vi "OPC Read Bool Variables.vi"() -> ()   [LabVIEW 2016]
uses:
  Architecture/Queue Management/ARC_Queue Valid.vi
panel:
  out "本地/远程":bool
  out "主电机准备好":bool
  out "主电机故障":bool
  out "主电机运行":bool
  out "变频器合闸":bool
  in  "Caller":string
  out "介质阀":bool
  out "增压1":bool
  out "排气1":bool
  out "进介质2":bool
  out "进介质1":bool
  out "增压2":bool
  out "排气2":bool
  out "调节阀电源":bool
  out "流量计电源":bool
  out "急停":bool
  out "容器间":bool
  out "球阀开":bool
  out "球阀关":bool
  out "油冷机故障":bool
  out "油冷机运行":bool
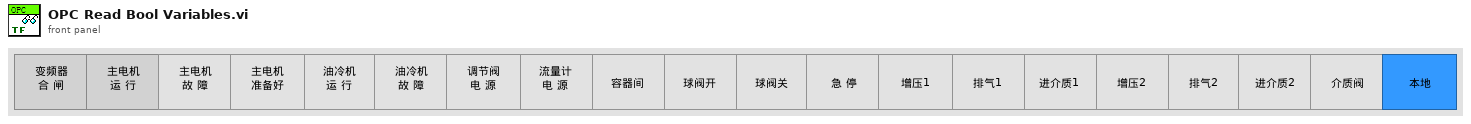
[diagram p1: front panel]
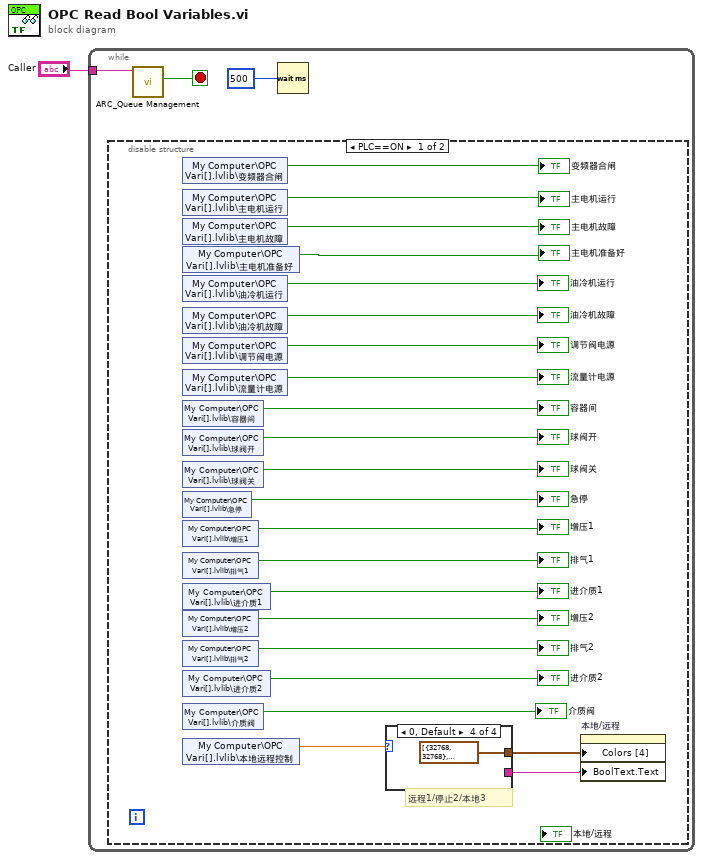
[diagram p0: block diagram]
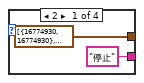
[diagram p2: hidden frame]
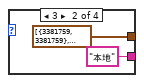
[diagram p3: hidden frame]
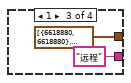
[diagram p4: hidden frame]
diagram:
  n1 = while {
    tunnel: "Caller" -> [w4]
    stop <- w2 stop-if-true
    n2 = disable-structure shown="PLC==ON" {
      frame condition #0 (active) {
        # "远程1/停止2/本地3"
        n3 = shared-variable "My Computer\\OPC Vari[].lvlib\\变频器合闸"() -> (→"变频器合闸":bool)  [unwired: 1 in, 1 out]
        n4 = shared-variable "My Computer\\OPC Vari[].lvlib\\主电机运行"() -> (→"主电机运行":bool)  [unwired: 1 in, 1 out]
        n5 = shared-variable "My Computer\\OPC Vari[].lvlib\\主电机故障"() -> (→"主电机故障":bool)  [unwired: 1 in, 1 out]
        n6 = shared-variable "My Computer\\OPC Vari[].lvlib\\主电机准备好"() -> (→"主电机准备好":bool)  [unwired: 1 in, 1 out]
        n7 = shared-variable "My Computer\\OPC Vari[].lvlib\\油冷机运行"() -> (→"油冷机运行":bool)  [unwired: 1 in, 1 out]
        n8 = shared-variable "My Computer\\OPC Vari[].lvlib\\油冷机故障"() -> (→"油冷机故障":bool)  [unwired: 1 in, 1 out]
        n9 = shared-variable "My Computer\\OPC Vari[].lvlib\\调节阀电源"() -> (→"调节阀电源":bool)  [unwired: 1 in, 1 out]
        n10 = shared-variable "My Computer\\OPC Vari[].lvlib\\流量计电源"() -> (→"流量计电源":bool)  [unwired: 1 in, 1 out]
        n11 = shared-variable "My Computer\\OPC Vari[].lvlib\\容器间"() -> (→"容器间":bool)  [unwired: 1 in, 1 out]
        n12 = shared-variable "My Computer\\OPC Vari[].lvlib\\球阀开"() -> (→"球阀开":bool)  [unwired: 1 in, 1 out]
        n13 = shared-variable "My Computer\\OPC Vari[].lvlib\\球阀关"() -> (→"球阀关":bool)  [unwired: 1 in, 1 out]
        n14 = shared-variable "My Computer\\OPC Vari[].lvlib\\急停"() -> (→"急停":bool)  [unwired: 1 in, 1 out]
        n15 = shared-variable "My Computer\\OPC Vari[].lvlib\\增压1"() -> (→"增压1":bool)  [unwired: 1 in, 1 out]
        n16 = shared-variable "My Computer\\OPC Vari[].lvlib\\排气1"() -> (→"排气1":bool)  [unwired: 1 in, 1 out]
        n17 = shared-variable "My Computer\\OPC Vari[].lvlib\\进介质1"() -> (→"进介质1":bool)  [unwired: 1 in, 1 out]
        n18 = shared-variable "My Computer\\OPC Vari[].lvlib\\增压2"() -> (→"增压2":bool)  [unwired: 1 in, 1 out]
        n19 = shared-variable "My Computer\\OPC Vari[].lvlib\\排气2"() -> (→"排气2":bool)  [unwired: 1 in, 1 out]
        n20 = shared-variable "My Computer\\OPC Vari[].lvlib\\进介质2"() -> (→"进介质2":bool)  [unwired: 1 in, 1 out]
        n21 = shared-variable "My Computer\\OPC Vari[].lvlib\\介质阀"() -> (→"介质阀":bool)  [unwired: 1 in, 1 out]
        n22 = shared-variable "My Computer\\OPC Vari[].lvlib\\本地远程控制"() -> (w11:sgl)  [unwired: 1 in, 1 out]
        n23 = case shown="0, Default" w11 {
          tunnel: ["停止" "本地" "远程" _] -> w5
          tunnel: [cluster{u32, u32}[] [{16774930, 16774930}, {7864153, 7864153}, {8354569, 8354569}, {806656, 3899180}] ("颜色[4]") cluster{u32, u32}[] [{3381759, 3381759}, {7864153, 7864153}, {1657983, 1657983}, {806656, 3899180}] ("颜色[4] 3") cluster{u32, u32}[] [{6618880, 6618880}, {7864153, 7864153}, {3309312, 3309312}, {806656, 3899180}] ("颜色[4] 3") cluster{u32, u32}[] [{32768, 32768}, {7864153, 7864153}, {729344, 2185728}, {806656, 3899180}] ("颜色[4] 2")] -> w6
          frame 2 {
          }
          frame 3 {
          }
          frame 1 {
          }
          frame 0, Default {
          }
        }
        n24 = property on="本地/远程" class="Bool"("Colors [4]"=w6, "BoolText.Text"=w5) -> ()  [unwired: 2 in, 2 out]
      }
      frame condition #1 {
      }
    }
    n25 = call-poly "ARC_Queue Management.vi"("Queue Name(unamed)"=w4) -> ("Not Exist?"=w2:bool)  [unwired: 8 in, 2 out]
    n26 = Wait (ms)(milliseconds to wait=u32 500 ("等待时间（毫秒）")) -> ()  [unwired: 1 out]
  }
